vi "ReadBinData.vi"() -> ()   [LabVIEW 2015]
panel:
  out "double precision float":dbl[](array[numeric])
  out "floor(x/y)":i64
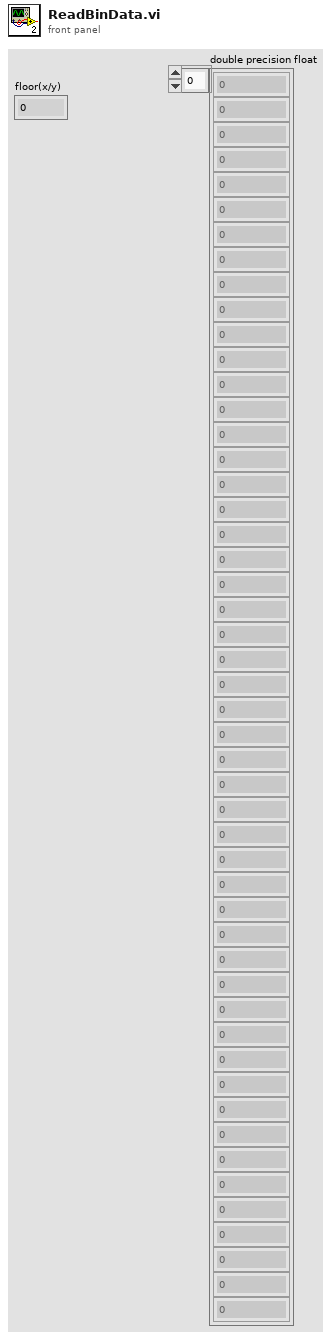
[diagram p1: front panel]
types:
  T1 = enum16{"big-endian, network order", "native, host order", "little-endian"}
  T2 = enum16{"open", "replace", "create", "open or create", "replace or create", "replace or create with confirmation"}
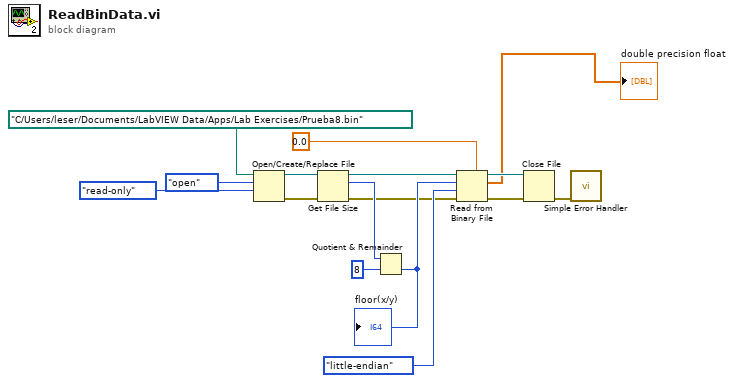
[diagram p0: block diagram]
diagram:
  n1 = Open/Create/Replace File(file path (use dialog)=path "C:/Users/leser/Documents/LabVIEW Data/Apps/Lab Exercises/Prueba8.bin" ("file (use dialog)"), operation (0:open)=T2."open", access (0:read/write)=enum16{"read/write", "read-only", "write-only"}."read-only") -> (refnum out=w9:refnum<file>, error out=w10:errorcluster)  [unwired: 3 in, 1 out]
  n2 = Get File Size(file=w9, error in=w10) -> (refnum out=w3:refnum<file>, size (in bytes)=w8:i64, 0:w4:errorcluster)
  n3 = Quotient & Remainder(x=w8, y=i64 8) -> (floor(x/y)=w6:i64)  [unwired: 1 out]
  "floor(x/y)" <- w6
  n4 = Read from Binary File(5:0.0, 8:w4, 9:T1."little-endian" ("byte order (0:big-endian, network order)"), 10:w6, 11:w3) -> (0:w12:errorcluster, 2:→"double precision float":dbl[], 3:w13:refnum<file>)  [unwired: 1 in, 1 out]
  n5 = Close File(refnum=w13, error in=w12) -> (error out=w11:errorcluster)  [unwired: 1 out]
  n6 = call <vilib>:"Simple Error Handler.vi"("error in (no error)"=w11) -> ()  [unwired: 4 in, 5 out]
